vi "conv[U8].vi"   [LabVIEW 2023]
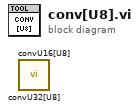
[diagram p0: block diagram]
diagram:
  n1 = call "convU32[U8].vi"() -> ()  [unwired: 2 in, 1 out]
  n2 = call "convU16[U8].vi"() -> ()  [unwired: 2 in, 1 out]
